vi "MGI RWA Remove EOLs and Slashes.vi"(8 "error in (no error)":errorcluster, 9 "Format String":string) -> (0 "error out":errorcluster, 1 "Format String without \\n":string)   [LabVIEW 2020]
doc: "Modify the format string to remove any \\n, \\r, or \\.\n\nOutput a warning if any characters are removed.\n\nAuthored by Shawn Walpole\nsupport@mooregoodideas.com\nwww.mooregoodideas.com\n\nCopyright (c) 2010, Moore Good Ideas, Inc.\n\nAll rights reserved.\n\nRedistribution and use in source and binary forms, with or without modification, are permitted provided that the following conditions are met:\n\n * Redistributions of source code must retain the above copyright notice, this list of conditions and the following disclaimer.\n * Redistributions in binary form must reproduce the above copyright notice, this list of conditions and the following disclaimer in the documentation and/or other materials provided with the distribution.\n * Neither the name of Moore Good Ideas, Inc. nor the names of its contributors may be used to endorse or promote products derived from this software without specific prior written permission.\n\nTHIS SOFTWARE IS PROVIDED BY THE COPYRIGHT HOLDERS AND CONTRIBUTORS \"AS IS\" AND ANY EXPRESS OR IMPLIED WARRANTIES, INCLUDING, BUT NOT LIMITED TO, THE IMPLIED WARRANTIES OF MERCHANTABILITY AND FITNESS FOR A PARTICULAR PURPOSE ARE DISCLAIMED. IN NO EVENT SHALL THE COPYRIGHT OWNER OR CONTRIBUTORS BE LIABLE FOR ANY DIRECT, INDIRECT, INCIDENTAL, SPECIAL, EXEMPLARY, OR CONSEQUENTIAL DAMAGES (INCLUDING, BUT NOT LIMITED TO, PROCUREMENT OF SUBSTITUTE GOODS OR SERVICES; LOSS OF USE, DATA, OR PROFITS; OR BUSINESS INTERRUPTION) HOWEVER CAUSED AND ON ANY THEORY OF LIABILITY, WHETHER IN CONTRACT, STRICT LIABILITY, OR TORT (INCLUDING NEGLIGENCE OR OTHERWISE) ARISING IN ANY WAY OUT OF THE USE OF THIS SOFTWARE, EVEN IF ADVISED OF THE POSSIBILITY OF SUCH DAMAGE."
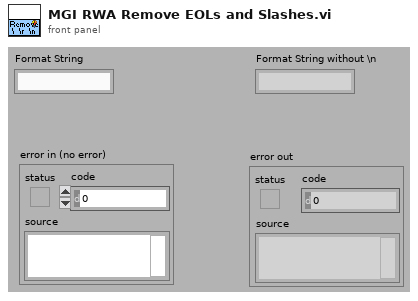
[diagram p1: front panel]
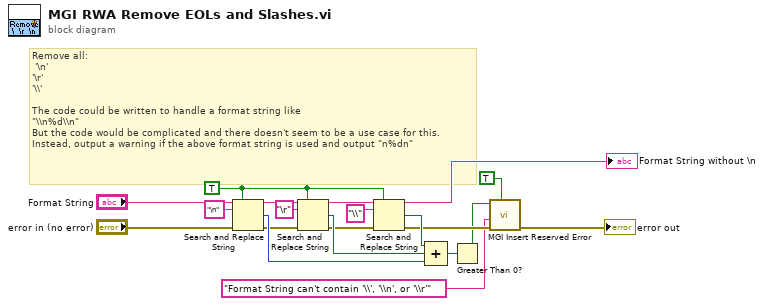
[diagram p0: block diagram]
diagram:
  w15 = TRUE ("replace all? (F)")
  # "Remove all:\n '\\n'\n'\\r'\n'\\\\'\n\nThe code could be written to handle a format string like\n\"\\\\n%d\\\\n\"\nBut the code would be complicated and there doesn't seem to be a use case for this.\nInstead, output a warning if the above format string is used and output \"n%dn\""
  n1 = Search and Replace String(replace all?=w15, input string="Format String", search string="\n", error in="error in (no error)") -> (result string=w19:string, number of replacements=w11:i32, error out=w10:errorcluster)  [unwired: 4 in, 1 out]
  n2 = Search and Replace String(replace all?=w15, input string=w19, search string="\r", error in=w10) -> (result string=w16:string, number of replacements=w12:i32, error out=w8:errorcluster)  [unwired: 4 in, 1 out]
  n3 = Search and Replace String(replace all?=w15, input string=w16, search string="\\", error in=w8) -> (result string=→"Format String without \\n":string, number of replacements=w13:i32, error out=w6:errorcluster)  [unwired: 4 in, 1 out]
  n4 = Compound Arithmetic op=ADD(w13, w12, w11) -> (w4:i32)
  n5 = Greater Than 0?(x=w4) -> (x > 0?=w3:bool)
  n6 = call "MGI Insert Reserved Error.vi"("Insert as Warning? (False: Insert as Error)"=TRUE, "Error In"=w6, "Error Description"="Format String can't contain '\\', '\\n', or '\\r'", "Error? (T)"=w3) -> ("Error Out"=→"error out":errorcluster)  [unwired: 7 in]
